vi "Read SerialData.vi"(8 "error in (no error)":errorcluster, 11 "PAS Data in":refnum<class "PAS Data.lvclass">) -> (0 "error out":errorcluster, 2 "SerialData":refnum<class "Data.lvclass">[](array[class]), 3 "PAS Data out":refnum<class "PAS Data.lvclass">)   [LabVIEW 2014]
uses:
  PAS Data.lvclass
  Data/Data.lvclass
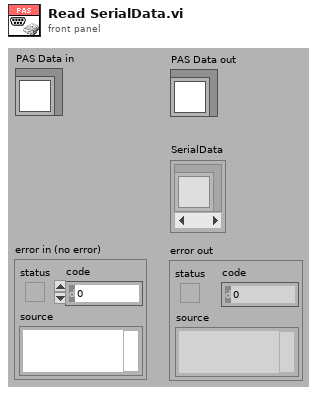
[diagram p1: front panel]
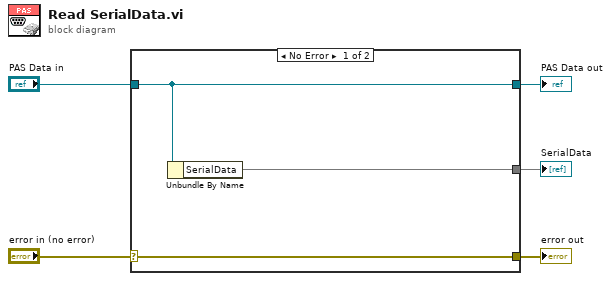
[diagram p0: block diagram]
diagram:
  n1 = case shown="No Error" "error in (no error)" {
    selector: "error in (no error)" -> [w8 w9]
    tunnel: [w8 w9] -> w4
    tunnel: [w7 w10] -> w2
    tunnel: "PAS Data in" -> [w7 w10]
    tunnel: [w6 _] -> w1
    frame No Error {
      n2 = Unbundle By Name(w7) -> ("SerialData"=w6)
    }
    frame Error {
    }
  }
  "error out" <- w4
  "PAS Data out" <- w2
  "SerialData" <- w1
